vi "Global 1.vi"() -> ()   [LabVIEW 2020]
panel:
  out "GlblSTOP":bool
  in  "Juhuarv2":dbl
  in  "Juhuarv1":dbl
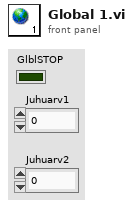
[diagram p1: front panel]
diagram:
